vi "PicoReadPicoMultiBuffers.vi"(1 "enabled array":i16[](array[numeric]), 2 "Buffer and Transfer Settings":T3={"startIndex"=0, "Samples"=1000000, "Down Sample Ratio"=1, "Down-Sample Mode"=2147483648} {"Down-Sample Mode" items=["None"=2147483648, "Aggregate"=1, "Decimate"=2, "Average"=4]; "Down Sample Ratio" step=1; "Samples" format="%_6p"}, 3 "Variant":string, 5 "Data Pointers":T1, 9 "No of Buffers":i32=1, 11 "error in (no error)":errorcluster) -> (6 "MultiBuffers (Max or non-aggregated)":T2(array[cluster]), 8 "Min Buffers":T2(array[cluster]), 15 "error out":errorcluster)   [LabVIEW 2010]
doc: "Read data from Picodata buffers for Block and 6000a streaming examples"
uses:
  PicoBuffers.ctl
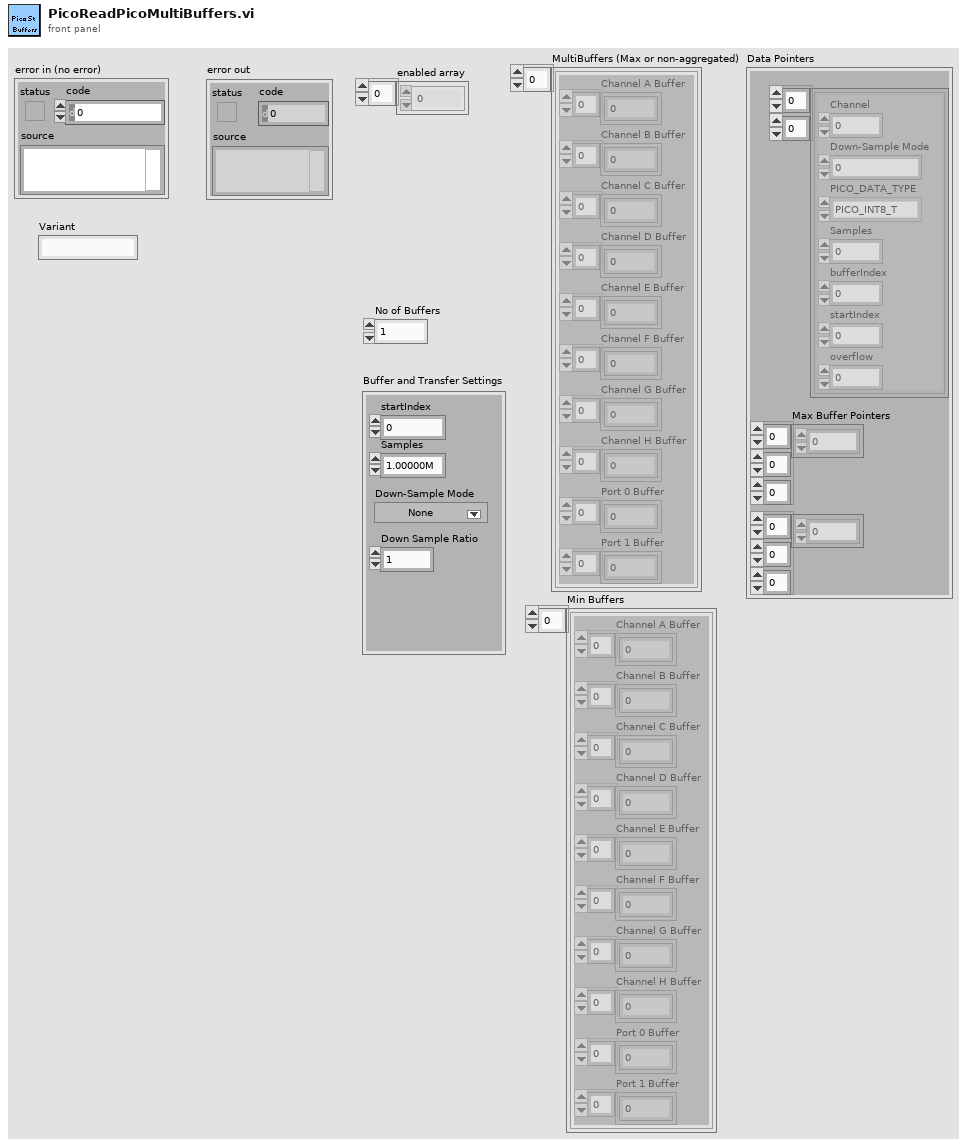
[diagram p1: front panel]
types:
  T1 = typedef "PicoBuffers.ctl" = cluster{"Max Buffer Pointers":u64[][][], "Min Buffer Pointers":u64[][][], "StreamingDataInfo":cluster{"Channel":u32, "Down-Sample Mode":u32, "PICO_DATA_TYPE":enum32{"PICO_INT8_T", "PICO_INT16_T", "PICO_INT32_T", "PICO_UINT32_T", "PICO_INT64_T", ""}, "Samples":i32, "bufferIndex":u64, "startIndex":i32, "overflow":i16}[][]}
  T2 = cluster{"Channel A Buffer":i16[], "Channel B Buffer":i16[], "Channel C Buffer":i16[], "Channel D Buffer":i16[], "Channel E Buffer":i16[], "Channel F Buffer":i16[], "Channel G Buffer":i16[], "Channel H Buffer":i16[], "Port 0 Buffer":i16[], "Port 1 Buffer":i16[]}[]
  T3 = cluster{"startIndex":u64, "Samples":u64, "Down Sample Ratio":u64, "Down-Sample Mode":u32}
  T4 = cluster{"Channel A Buffer":i16[], "Channel B Buffer":i16[], "Channel C Buffer":i16[], "Channel D Buffer":i16[], "Channel E Buffer":i16[], "Channel F Buffer":i16[], "Channel G Buffer":i16[], "Channel H Buffer":i16[], "Port 0 Buffer":i16[], "Port 1 Buffer":i16[]}
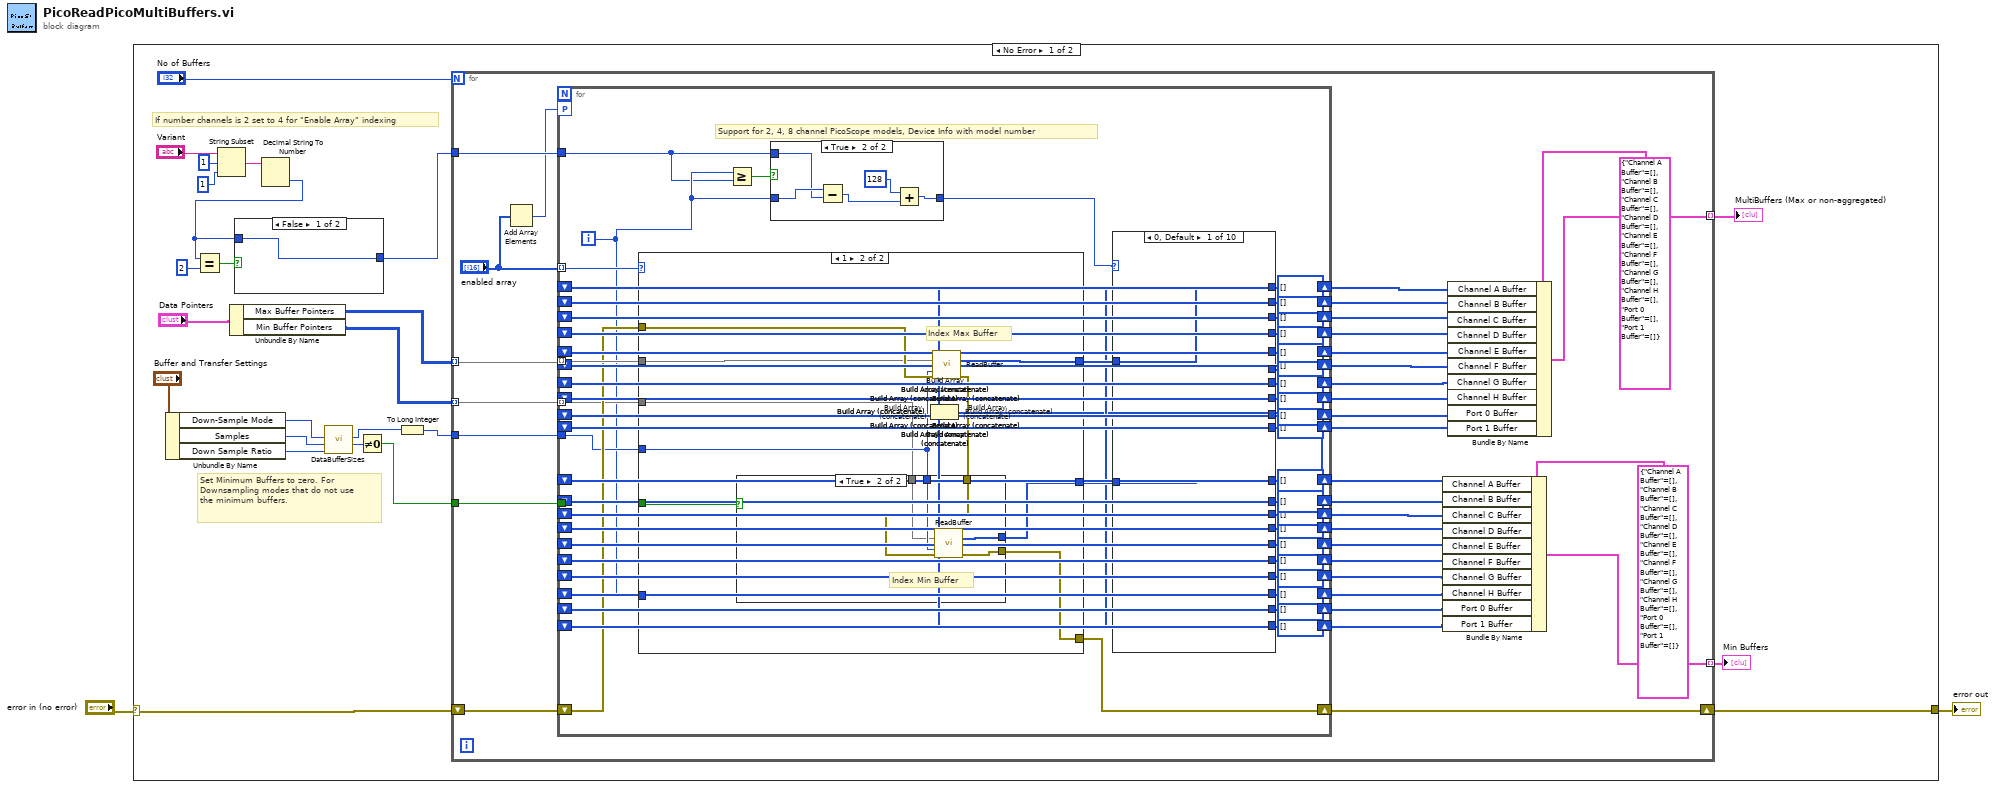
[diagram p0: block diagram]
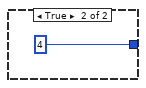
[diagram p2: hidden frame]
diagram:
  n1 = case shown="No Error" "error in (no error)" {
    selector: "error in (no error)" -> [w24 w197]
    tunnel: [w26 w197] -> w1
    frame No Error {
      # "If number channels is 2 set to 4 for \"Enable Array\" indexing"
      # "Set Minimum Buffers to zero. For Downsampling modes that do not use the minimum buffers."
      n2 = Unbundle By Name("Buffer and Transfer Settings") -> ("Down-Sample Mode"=w22:u32, "Samples"=w21:u64, "Down Sample Ratio"=w23:u64)
      n3 = String Subset(string="Variant", offset (0)=1, length (rest)=1 ("length (rest)")) -> (substring=w7:string)
      n4 = Unbundle By Name("Data Pointers") -> ("Max Buffer Pointers"=w12:u64[][][], "Min Buffer Pointers"=w11:u64[][][])
      n5 = Decimal String To Number(string=w7) -> (number=w4:i32)  [unwired: 2 in, 1 out]
      n6 = Equal?(x=w4, y=2 ("Number of channels")) -> (x = y?=w10:bool)
      n7 = case shown="False" w10 {
        tunnel: [w27 4 ("Number of channels")] -> w8
        tunnel: w4 -> [w27 _]
        frame False {
        }
        frame True {
        }
      }
      n8 = call "DataBufferSizes.vi"("Down Sample Ratio"=w23, "Number of Samples"=w21, "Down-Sample Mode"=w22) -> ("min Buffer Size"=w19:i32, "Max Buffer Size"=w15:i32)  [unwired: 7 in]
      n9 = Not Equal To 0?(x=w19) -> (x != 0?=w20:bool)
      n10 = To Long Integer(number=w15) -> (32bit integer=w18:i32)
      n11 = for {
        N: "No of Buffers" -> [_]
        tunnel: [w79] -> w14 mode=indexing
        tunnel: [w78] -> w16 mode=indexing
        tunnel: w20 -> [w66]
        tunnel: w18 -> [w64]
        shift-right: [w81] -> w26
        shift-left: w24 -> [w80]
        tunnel: w12 -> [w63] mode=indexing
        tunnel: w11 -> [w52] mode=indexing
        tunnel: w8 -> [w51]
        n12 = Add Array Elements(numeric array="enabled array") -> (sum=w49:i16)
        n13 = for {
          tunnel: "enabled array" -> [w153] mode=indexing
          tunnel: w63 -> [w154] mode=indexing
          shift-right: [w152] -> w81
          shift-left: w80 -> [w151]
          tunnel: w64 -> [w137]
          tunnel: w66 -> [w136]
          tunnel: w52 -> [w126] mode=indexing
          tunnel: w51 -> [w122]
          workers-P: w49 -> [_]
          shift-right: [w120] -> w77
          shift-left: i16[] [] ("Output Array") -> [w121]
          shift-right: [w118] -> w76
          shift-left: i16[] [] ("Output Array") -> [w119]
          shift-right: [w116] -> w75
          shift-left: i16[] [] ("Output Array") -> [w117]
          shift-right: [w114] -> w74
          shift-left: i16[] [] ("Output Array") -> [w115]
          shift-right: [w112] -> w73
          shift-left: i16[] [] ("Output Array") -> [w113]
          shift-right: [w110] -> w72
          shift-left: i16[] [] ("Output Array") -> [w111]
          shift-right: [w108] -> w65
          shift-left: i16[] [] ("Output Array") -> [w109]
          shift-right: [w106] -> w71
          shift-left: i16[] [] ("Output Array") -> [w107]
          shift-right: [w104] -> w70
          shift-left: i16[] [] ("Output Array") -> [w105]
          shift-right: [w102] -> w69
          shift-left: i16[] [] ("Output Array") -> [w103]
          shift-right: [w100] -> w68
          shift-left: i16[] [] ("Output Array") -> [w101]
          shift-right: [w98] -> w67
          shift-left: i16[] [] ("Output Array") -> [w99]
          shift-right: [w96] -> w60
          shift-left: i16[] [] ("Output Array") -> [w97]
          shift-right: [w94] -> w59
          shift-left: i16[] [] ("Output Array") -> [w95]
          shift-right: [w92] -> w58
          shift-left: i16[] [] ("Output Array") -> [w93]
          shift-right: [w90] -> w57
          shift-left: i16[] [] ("Output Array") -> [w91]
          shift-right: [w88] -> w56
          shift-left: i16[] [] ("Output Array") -> [w89]
          shift-right: [w86] -> w55
          shift-left: i16[] [] ("Output Array") -> [w87]
          shift-right: [w84] -> w54
          shift-left: i16[] [] ("Output Array") -> [w85]
          shift-right: [w82] -> w53
          shift-left: i16[] [] ("Output Array") -> [w83]
          i -> [w123]
          # "Support for 2, 4, 8 channel PicoScope models, Device Info with model number"
          n14 = case shown="1" w153 {
            tunnel: w154 -> [_ w183]
            tunnel: w123 -> [_ _]
            tunnel: [_ w190] -> w150
            tunnel: [_ w189] -> w149
            tunnel: w151 -> [w181 w188]
            tunnel: [w181 w186] -> w152
            tunnel: w137 -> [_ w184]
            tunnel: w136 -> [_ w185]
            tunnel: w126 -> [_ w182]
            frame 0, Default {
            }
            frame 1 {
              # "Index Max Buffer"
              n15 = call "ReadBuffer.vi"("Pointer and BufferSize"=w183, "Buffer size"=w184, "error in (no error)"=w188) -> ("Output Array"=w190:i16[], "error out"=w187:errorcluster)  [unwired: 11 in]
              n16 = case shown="True" w185 {
                tunnel: [_ w196] -> w189
                tunnel: w187 -> [w191 w195]
                tunnel: [w191 w194] -> w186
                tunnel: w184 -> [_ w193]
                tunnel: w182 -> [_ w192]
                frame False {
                }
                frame True {
                  # "Index Min Buffer"
                  n17 = call "ReadBuffer.vi"("Pointer and BufferSize"=w192, "Buffer size"=w193, "error in (no error)"=w195) -> ("Output Array"=w196:i16[], "error out"=w194:errorcluster)  [unwired: 11 in]
                }
              }
            }
          }
          n18 = Greater Or Equal?(x=w123, y=w122) -> (x >= y?=w125:bool)
          n19 = case shown="True" w125 {
            tunnel: w123 -> [w155 w157]
            tunnel: [w155 w159] -> w124
            tunnel: w122 -> [_ w156]
            frame False {
            }
            frame True {
              n20 = Subtract(x=w157, y=w156) -> (x-y=w158:i32)
              n21 = Add(x=128, y=w158) -> (x+y=w159:i32)
            }
          }
          n22 = case shown="0, Default" w124 {
            tunnel: w150 -> [w162 w164 w166 w168 w170 w172 w174 w176 w178 w180]
            tunnel: [w162 _ _ _ _ _ _ _ _ _] -> w135
            tunnel: [_ w164 _ _ _ _ _ _ _ _] -> w142
            tunnel: [_ _ w166 _ _ _ _ _ _ _] -> w141
            tunnel: [_ _ _ w168 _ _ _ _ _ _] -> w140
            tunnel: [_ _ _ _ w170 _ _ _ _ _] -> w139
            tunnel: [_ _ _ _ _ w172 _ _ _ _] -> w138
            tunnel: w149 -> [w161 w163 w165 w167 w169 w171 w173 w175 w177 w179]
            tunnel: [w161 _ _ _ _ _ _ _ _ _] -> w148
            tunnel: [_ w163 _ _ _ _ _ _ _ _] -> w147
            tunnel: [_ _ w165 _ _ _ _ _ _ _] -> w146
            tunnel: [_ _ _ w167 _ _ _ _ _ _] -> w145
            tunnel: [_ _ _ _ w169 _ _ _ _ _] -> w144
            tunnel: [_ _ _ _ _ w171 _ _ _ _] -> w143
            tunnel: [_ _ _ _ _ _ w174 _ _ _] -> w134
            tunnel: [_ _ _ _ _ _ w173 _ _ _] -> w133
            tunnel: [_ _ _ _ _ _ _ w176 _ _] -> w132
            tunnel: [_ _ _ _ _ _ _ w175 _ _] -> w131
            tunnel: [_ _ _ _ _ _ _ _ w178 _] -> w130
            tunnel: [_ _ _ _ _ _ _ _ w177 _] -> w129
            tunnel: [_ _ _ _ _ _ _ _ _ w180] -> w128
            tunnel: [_ _ _ _ _ _ _ _ _ w179] -> w127
            frame 0, Default {
            }
            frame 1 {
            }
            frame 2 {
            }
            frame 3 {
            }
            frame 4 {
            }
            frame 5 {
            }
            frame 6 {
            }
            frame 7 {
            }
            frame 128 {
            }
            frame 129 {
            }
          }
          n23 = Build Array (concatenate)(w83, w127) -> (w82:i16[])
          n24 = Build Array (concatenate)(w85, w128) -> (w84:i16[])
          n25 = Build Array (concatenate)(w87, w129) -> (w86:i16[])
          n26 = Build Array (concatenate)(w89, w130) -> (w88:i16[])
          n27 = Build Array (concatenate)(w91, w131) -> (w90:i16[])
          n28 = Build Array (concatenate)(w93, w132) -> (w92:i16[])
          n29 = Build Array (concatenate)(w95, w133) -> (w94:i16[])
          n30 = Build Array (concatenate)(w97, w134) -> (w96:i16[])
          n31 = Build Array (concatenate)(w99, w138) -> (w98:i16[])
          n32 = Build Array (concatenate)(w101, w139) -> (w100:i16[])
          n33 = Build Array (concatenate)(w103, w140) -> (w102:i16[])
          n34 = Build Array (concatenate)(w105, w141) -> (w104:i16[])
          n35 = Build Array (concatenate)(w107, w142) -> (w106:i16[])
          n36 = Build Array (concatenate)(w109, w135) -> (w108:i16[])
          n37 = Build Array (concatenate)(w111, w143) -> (w110:i16[])
          n38 = Build Array (concatenate)(w113, w144) -> (w112:i16[])
          n39 = Build Array (concatenate)(w115, w145) -> (w114:i16[])
          n40 = Build Array (concatenate)(w117, w146) -> (w116:i16[])
          n41 = Build Array (concatenate)(w119, w147) -> (w118:i16[])
          n42 = Build Array (concatenate)(w121, w148) -> (w120:i16[])
        }
        n43 = Bundle By Name(cluster=T4 {"Channel A Buffer"=[], "Channel B Buffer"=[], "Channel C Buffer"=[], "Channel D Buffer"=[], "Channel E Buffer"=[], "Channel F Buffer"=[], "Channel G Buffer"=[], "Channel H Buffer"=[], "Port 0 Buffer"=[], "Port 1 Buffer"=[]} ("input cluster"), "Channel A Buffer"=w77, "Channel B Buffer"=w76, "Channel C Buffer"=w75, "Channel D Buffer"=w74, "Channel E Buffer"=w73, "Channel F Buffer"=w72, "Channel G Buffer"=w59, "Channel H Buffer"=w57, "Port 0 Buffer"=w55, "Port 1 Buffer"=w53) -> (w79:T4)
        n44 = Bundle By Name(cluster=T4 {"Channel A Buffer"=[], "Channel B Buffer"=[], "Channel C Buffer"=[], "Channel D Buffer"=[], "Channel E Buffer"=[], "Channel F Buffer"=[], "Channel G Buffer"=[], "Channel H Buffer"=[], "Port 0 Buffer"=[], "Port 1 Buffer"=[]} ("input cluster"), "Channel A Buffer"=w65, "Channel B Buffer"=w71, "Channel C Buffer"=w70, "Channel D Buffer"=w69, "Channel E Buffer"=w68, "Channel F Buffer"=w67, "Channel G Buffer"=w60, "Channel H Buffer"=w58, "Port 0 Buffer"=w56, "Port 1 Buffer"=w54) -> (w78:T4)
      }
      "MultiBuffers (Max or non-aggregated)" <- w16
      "Min Buffers" <- w14
    }
    frame Error {
    }
  }
  "error out" <- w1
